vi "test_input_format.vi"() -> ()   [LabVIEW 2025]
panel:
  in  "factor":u16
  in  "val":fxp<+/-,18,1>
  out "Array":fxp<+/-,32,14>[](array[numeric])
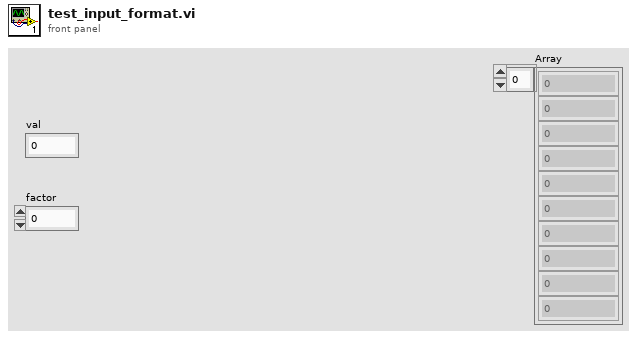
[diagram p1: front panel]
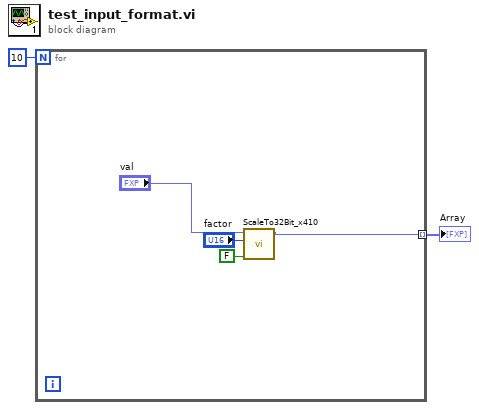
[diagram p0: block diagram]
diagram:
  n1 = for {
    N: 10 -> [_]
    tunnel: [w6] -> w1 mode=indexing
    n2 = call "ScaleTo32Bit_x410.vi"("valid in"=FALSE, "factor"="factor", "val"="val") -> ("32 bit fxp"=w6:fxp<+/-,32,14>)  [unwired: 7 in, 1 out]
  }
  "Array" <- w1
